vi "log analysis_gps.vi"() -> ()   [LabVIEW 2019] (continued)
8.2238,22.3000,0.0031,0.0013,-0.0034,-0.411270923,-0.605029312,287.914838543,0.2104,0.1573,0.2657,0.0344,0.0343,0.0312,0.0795,0.0805,4.9275,0f000005,0*6d07f4f4\n\t", "INSPVAXA,USB3,0,44.0,FINESTEERING,2107,283111.250,02000000,471d,15824;INS_ALIGNMENT_COMPLETE,INS_RTKFIXED,37.37108787798,126.72336901339,8.2237,22.3000,0.0035,0.0008,-0.0027,-0.411014484,-0.606801614,287.916144015,0.2104,0.1572,0.2653,0.0344,0.0343,0.0312,0.0795,0.0805,4.9290,0f000005,0*17fda63e\n\t", "INSPVAXA,USB3,0,46.5,FINESTEERING,2107,283112.250,02000000,471d,15824;INS_ALIGNMENT_COMPLETE,INS_RTKFIXED,37.37108788668,126.72336900523,8.2241,22.3000,0.0049,-0.0005,-0.0016,-0.408777501,-0.612185293,287.914677114,0.2103,0.1572,0.2649,0.0344,0.0343,0.0312,0.0795,0.0805,4.9305,0f000005,0*82ade194\n\t", "INSPVAXA,USB3,0,46.5,FINESTEERING,2107,283112.750,02000000,471d,15824;INS_ALIGNMENT_COMPLETE,INS_RTKFIXED,37.37108788778,126.72336899951,8.2242,22.3000,0.0047,-0.0009,-0.0019,-0.409122282,-0.611972311,287.914890224,0.2103,0.1572,0.2649,0.0344,0.0343,0.0312,0.0795,0.0805,4.9305,0f000005,0*c3a4b162\n\t", "INSPVAXA,USB3,0,48.5,FINESTEERING,2107,283113.250,02000000,471d,15824;INS_ALIGNMENT_COMPLETE,INS_RTKFIXED,37.37108788861,126.72336899425,8.2243,22.3000,0.0050,-0.0013,-0.0019,-0.410508140,-0.611024198,287.914176571,0.2103,0.1572,0.2646,0.0344,0.0343,0.0312,0.0795,0.0805,4.9321,0f000005,0*87d2d5b6\n\t", "INSPVAXA,USB3,0,48.5,FINESTEERING,2107,283113.750,02000000,471d,15824;INS_ALIGNMENT_COMPLETE,INS_RTKFIXED,37.37108789363,126.72336898840,8.2244,22.3000,0.0063,-0.0021,-0.0017,-0.411022705,-0.609051513,287.913579305,0.2103,0.1572,0.2646,0.0344,0.0343,0.0312,0.0795,0.0805,4.9321,0f000005,0*35e79e67\n\t", "INSPVAXA,USB3,0,47.0,FINESTEERING,2107,283114.250,02000000,471d,15824;INS_ALIGNMENT_COMPLETE,INS_RTKFIXED,37.37108789523,126.72336898295,8.2245,22.3000,0.0061,-0.0024,-0.0023,-0.410389175,-0.608679796,287.908436695,0.2102,0.1572,0.2643,0.0344,0.0343,0.0312,0.0795,0.0805,4.9336,0f000005,0*e900128e\n\t", "INSPVAXA,USB3,0,47.0,FINESTEERING,2107,283114.750,02000000,471d,15824;INS_ALIGNMENT_COMPLETE,INS_RTKFIXED,37.37108789043,126.72336897889,8.2245,22.3000,0.0054,-0.0027,-0.0027,-0.410079836,-0.608000188,287.907030910,0.2102,0.1572,0.2643,0.0344,0.0343,0.0312,0.0795,0.0805,4.9336,0f000005,0*f5aa2bf4\n\t", "INSPVAXA,USB3,0,46.0,FINESTEERING,2107,283115.250,02000000,471d,15824;INS_ALIGNMENT_COMPLETE,INS_RTKFIXED,37.37108788786,126.72336897498,8.2245,22.3000,0.0055,-0.0029,-0.0021,-0.409736809,-0.602715261,287.905938302,0.2101,0.1572,0.2640,0.0344,0.0343,0.0312,0.0795,0.0805,4.9352,0f000005,0*b8856e6c\n\t", "INSPVAXA,USB3,0,46.0,FINESTEERING,2107,283115.750,02000000,471d,15824;INS_ALIGNMENT_COMPLETE,INS_RTKFIXED,37.37108788493,126.72336897577,8.2245,22.3000,0.0046,-0.0023,-0.0026,-0.410098984,-0.602405796,287.902959038,0.2101,0.1572,0.2640,0.0344,0.0343,0.0312,0.0795,0.0805,4.9352,0f000005,0*5724c76a\n\t", "INSPVAXA,USB3,0,48.5,FINESTEERING,2107,283117.250,02000000,471d,15824;INS_ALIGNMENT_COMPLETE,INS_RTKFIXED,37.37108787822,126.72336898248,8.2247,22.3000,0.0046,0.0006,-0.0022,-0.408932053,-0.597708499,287.898385765,0.2100,0.1572,0.2634,0.0344,0.0343,0.0312,0.0795,0.0805,4.9381,0f000005,0*450763d8\n\t", "INSPVAXA,USB3,0,51.5,FINESTEERING,2107,283118.750,02000000,471d,15824;INS_ALIGNMENT_COMPLETE,INS_RTKFIXED,37.37108787489,126.72336898888,8.2255,22.3000,0.0051,0.0006,-0.0004,-0.410553255,-0.597325999,287.895855349,0.2099,0.1572,0.2632,0.0344,0.0343,0.0312,0.0794,0.0805,4.9396,0f000005,0*531bbf8e\n\t", "INSPVAXA,USB3,0,49.0,FINESTEERING,2107,283119.750,02000000,471d,15824;INS_ALIGNMENT_COMPLETE,INS_RTKFIXED,37.37108788239,126.72336898736,8.2256,22.3000,0.0062,0.0005,-0.0005,-0.410245690,-0.596223685,287.896349306,0.2099,0.1572,0.2630,0.0344,0.0343,0.0312,0.0794,0.0805,4.9410,0f000005,0*aabca186\n\t", "INSPVAXA,USB3,0,47.5,FINESTEERING,2107,283120.250,02000000,471d,15824;INS_ALIGNMENT_COMPLETE,INS_RTKFIXED,37.37108788462,126.72336898711,8.2255,22.3000,0.0062,0.0002,-0.0014,-0.410019875,-0.596819628,287.894466218,0.2099,0.1572,0.2628,0.0344,0.0343,0.0312,0.0794,0.0805,4.9425,0f000005,0*feb71611\n\t", "INSPVAXA,USB3,0,47.5,FINESTEERING,2107,283121.250,02000000,471d,15824;INS_ALIGNMENT_COMPLETE,INS_RTKFIXED,37.37108788020,126.72336899019,8.2251,22.3000,0.0049,0.0012,-0.0017,-0.410504520,-0.596359600,287.895045223,0.2098,0.1572,0.2627,0.0344,0.0343,0.0312,0.0794,0.0805,4.9439,0f000005,0*861abdab\n\t", "INSPVAXA,USB3,0,48.0,FINESTEERING,2107,283122.250,02000000,471d,15824;INS_ALIGNMENT_COMPLETE,INS_RTKFIXED,37.37108788140,126.72336898679,8.2256,22.3000,0.0046,0.0003,-0.0020,-0.412214067,-0.597500472,287.894257245,0.2098,0.1572,0.2625,0.0344,0.0343,0.0312,0.0794,0.0805,4.9454,0f000005,0*41de74d7\n\t", "INSPVAXA,USB3,0,46.5,FINESTEERING,2107,283126.250,02000000,471d,15824;INS_ALIGNMENT_COMPLETE,INS_RTKFIXED,37.37108785781,126.72336899407,8.2263,22.3000,0.0034,0.0010,-0.0014,-0.405163325,-0.599911050,287.885200973,0.2098,0.1572,0.2620,0.0344,0.0343,0.0312,0.0794,0.0804,4.9511,0f000005,0*554930fc\n\t", "INSPVAXA,USB3,0,50.5,FINESTEERING,2107,283133.250,02008000,471d,15824;INS_ALIGNMENT_COMPLETE,INS_RTKFIXED,37.37108787441,126.72336901696,8.2251,22.3000,0.0051,0.0025,0.0013,-0.401038405,-0.592309574,287.886306258,0.2098,0.1572,0.2615,0.0344,0.0343,0.0312,0.0794,0.0804,4.9611,0f000005,0*3f736d45\n\t", "INSPVAXA,USB3,0,50.0,FINESTEERING,2107,283145.800,02000000,471d,15824;INS_ALIGNMENT_COMPLETE,INS_RTKFIXED,37.37108786440,126.72336901151,8.2210,22.3000,0.0034,-0.0002,0.0004,-0.408176107,-0.602369941,287.881922019,0.2098,0.1572,0.2612,0.0344,0.0343,0.0312,0.0794,0.0804,4.9785,0f000005,0*1b1c4bf8\n\t", "INSPVAXA,USB3,0,45.5,FINESTEERING,2107,283151.800,02000000,471d,15824;INS_ALIGNMENT_COMPLETE,INS_RTKFIXED,37.37108787046,126.72336898866,8.2212,22.3000,0.0033,0.0009,-0.0006,-0.404916149,-0.597406910,287.865620586,0.2099,0.1572,0.2612,0.0344,0.0343,0.0312,0.0793,0.0804,4.9878,0f000005,0*a5f125e6\n\t", "INSPVAXA,USB3,0,45.0,FINESTEERING,2107,283152.300,02000000,471d,15824;INS_ALIGNMENT_COMPLETE,INS_RTKFIXED,37.37108786806,126.72336899217,8.2208,22.3000,0.0029,0.0018,-0.0009,-0.404359469,-0.596798726,287.864856489,0.2099,0.1572,0.2612,0.0344,0.0343,0.0312,0.0793,0.0804,4.9892,0f000005,0*75438a82\n\t", "INSPVAXA,USB3,0,47.5,FINESTEERING,2107,283153.800,02000000,471d,15824;INS_ALIGNMENT_COMPLETE,INS_RTKFIXED,37.37108786600,126.72336899902,8.2205,22.3000,0.0026,0.0021,-0.0023,-0.403425682,-0.598266477,287.862635982,0.2098,0.1572,0.2612,0.0344,0.0343,0.0312,0.0793,0.0804,4.9906,0f000005,0*5c2a9c66\n\t", "INSPVAXA,USB3,0,49.0,FINESTEERING,2107,283155.800,02000000,471d,15824;INS_ALIGNMENT_COMPLETE,INS_RTKFIXED,37.37108786878,126.72336899361,8.2202,22.3000,0.0032,0.0004,-0.0022,-0.395795579,-0.599014783,287.862450492,0.2098,0.1572,0.2612,0.0344,0.0343,0.0312,0.0793,0.0804,4.9935,0f000005,0*f4cd5051\n\t", "INSPVAXA,USB3,0,46.5,FINESTEERING,2107,283156.300,02000000,471d,15824;INS_ALIGNMENT_COMPLETE,INS_RTKFIXED,37.37108786919,126.72336899093,8.2205,22.3000,0.0038,-0.0001,-0.0013,-0.396437672,-0.598313647,287.862503112,0.2098,0.1572,0.2612,0.0344,0.0343,0.0312,0.0793,0.0804,4.9950,0f000005,0*5aa32664\n\t", "INSPVAXA,USB3,0,46.5,FINESTEERING,2107,283156.800,02000000,471d,15824;INS_ALIGNMENT_COMPLETE,INS_RTKFIXED,37.37108787385,126.72336898941,8.2207,22.3000,0.0043,-0.0002,-0.0010,-0.392731293,-0.598638690,287.862042656,0.2098,0.1572,0.2612,0.0344,0.0343,0.0312,0.0793,0.0804,4.9950,0f000005,0*03d612e4\n\t", "INSPVAXA,USB3,0,51.0,FINESTEERING,2107,283157.300,02000000,471d,15824;INS_ALIGNMENT_COMPLETE,INS_RTKFIXED,37.37108787685,126.72336898846,8.2211,22.3000,0.0052,-0.0002,-0.0000,-0.390778583,-0.597437105,287.863000385,0.2098,0.1573,0.2612,0.0344,0.0343,0.0312,0.0793,0.0804,4.9965,0f000005,0*3bc0d928\n\t", "INSPVAXA,USB3,0,50.5,FINESTEERING,2107,283159.300,02000000,471d,15824;INS_ALIGNMENT_COMPLETE,INS_RTKFIXED,37.37108788569,126.72336899544,8.2223,22.3000,0.0068,0.0019,0.0013,-0.387086330,-0.593973069,287.861144002,0.2098,0.1573,0.2612,0.0344,0.0343,0.0312,0.0793,0.0803,4.9994,0f000005,0*0ed095af\n\t", "INSPVAXA,USB3,0,44.5,FINESTEERING,2107,283160.800,02000000,471d,15824;INS_ALIGNMENT_COMPLETE,INS_RTKFIXED,37.37108790025,126.72336900642,8.2224,22.3000,0.0087,0.0034,0.0012,-0.385305357,-0.593887975,287.861236180,0.2098,0.1573,0.2612,0.0344,0.0343,0.0312,0.0793,0.0803,5.0008,0f000005,0*a535fac5\n\t", "INSPVAXA,USB3,0,47.0,FINESTEERING,2107,283161.800,02000000,471d,15824;INS_ALIGNMENT_COMPLETE,INS_RTKFIXED,37.37108791058,126.72336901739,8.2224,22.3000,0.0091,0.0053,0.0008,-0.384677214,-0.593155644,287.863440186,0.2098,0.1573,0.2612,0.0344,0.0343,0.0312,0.0793,0.0803,5.0020,0f000005,0*15bd2f54\n\t", "INSPVAXA,USB3,0,49.0,FINESTEERING,2107,283162.300,02000000,471d,15824;INS_ALIGNMENT_COMPLETE,INS_RTKFIXED,37.37108791275,126.72336902289,8.2223,22.3000,0.0092,0.0053,0.0006,-0.383976052,-0.593983766,287.863552246,0.2098,0.1573,0.2612,0.0344,0.0343,0.0312,0.0793,0.0803,5.0033,0f000005,0*f7f4aafb\n\t", "INSPVAXA,USB3,0,49.0,FINESTEERING,2107,283162.800,02000000,471d,15824;INS_ALIGNMENT_COMPLETE,INS_RTKFIXED,37.37108791707,126.72336902756,8.2221,22.3000,0.0099,0.0052,0.0004,-0.383244439,-0.593582797,287.863703162,0.2098,0.1573,0.2612,0.0344,0.0343,0.0312,0.0793,0.0803,5.0033,0f000005,0*87119b1a\n\t", "INSPVAXA,USB3,0,50.0,FINESTEERING,2107,283163.300,02000000,471d,15824;INS_ALIGNMENT_COMPLETE,INS_RTKFIXED,37.37108791768,126.72336903031,8.2218,22.3000,0.0093,0.0052,-0.0002,-0.382087992,-0.594481290,287.864257970,0.2098,0.1573,0.2612,0.0344,0.0343,0.0312,0.0793,0.0803,5.0046,0f000005,0*64efd3fe\n\t", "INSPVAXA,USB3,0,50.0,FINESTEERING,2107,283163.800,02000000,471d,15824;INS_ALIGNMENT_COMPLETE,INS_RTKFIXED,37.37108791823,126.72336903544,8.2213,22.3000,0.0087,0.0054,-0.0002,-0.381855357,-0.594537838,287.865100598,0.2098,0.1573,0.2612,0.0344,0.0343,0.0312,0.0793,0.0803,5.0046,0f000005,0*eaa89ec3\n\t", "INSPVAXA,USB3,0,49.5,FINESTEERING,2107,283164.300,02000000,471d,15824;INS_ALIGNMENT_COMPLETE,INS_RTKFIXED,37.37108791762,126.72336903818,8.2211,22.3000,0.0096,0.0053,-0.0000,-0.380427968,-0.595358698,287.865754120,0.2100,0.1573,0.2613,0.0344,0.0343,0.0312,0.0793,0.0803,5.0060,0f000005,0*9eb07253\n\t", "INSPVAXA,USB3,0,49.5,FINESTEERING,2107,283164.800,02000000,471d,15824;INS_ALIGNMENT_COMPLETE,INS_RTKFIXED,37.37108792129,126.72336904200,8.2211,22.3000,0.0095,0.0050,0.0001,-0.381479450,-0.593246291,287.867192627,0.2100,0.1573,0.2613,0.0344,0.0343,0.0312,0.0793,0.0803,5.0060,0f000005,0*81097ed9\n\t", "INSPVAXA,USB3,0,48.5,FINESTEERING,2107,283165.300,02000000,471d,15824;INS_ALIGNMENT_COMPLETE,INS_RTKFIXED,37.37108792359,126.72336904372,8.2212,22.3000,0.0098,0.0050,0.0003,-0.382461437,-0.592905475,287.870739528,0.2103,0.1573,0.2614,0.0344,0.0343,0.0312,0.0793,0.0803,5.0073,0f000005,0*f350cda0\n\t", "INSPVAXA,USB3,0,48.5,FINESTEERING,2107,283165.800,02000000,471d,15824;INS_ALIGNMENT_COMPLETE,INS_RTKFIXED,37.37108792768,126.72336904655,8.2215,22.3000,0.0096,0.0053,0.0004,-0.381584283,-0.591456419,287.872579847,0.2103,0.1573,0.2614,0.0344,0.0343,0.0312,0.0793,0.0803,5.0073,0f000005,0*a9ef8806\n\t", "INSPVAXA,USB3,0,47.0,FINESTEERING,2107,283166.300,02000000,471d,15824;INS_ALIGNMENT_COMPLETE,INS_RTKFIXED,37.37108793024,126.72336904905,8.2215,22.3000,0.0104,0.0057,0.0003,-0.382222726,-0.592164318,287.872646767,0.2105,0.1573,0.2615,0.0344,0.0343,0.0312,0.0793,0.0803,5.0087,0f000005,0*6f064ef0\n\t", "INSPVAXA,USB3,0,47.0,FINESTEERING,2107,283166.800,02000000,471d,15824;INS_ALIGNMENT_COMPLETE,INS_RTKFIXED,37.37108793672,126.72336905212,8.2216,22.3000,0.0107,0.0058,0.0001,-0.380800259,-0.589429313,287.874913684,0.2105,0.1573,0.2615,0.0344,0.0343,0.0312,0.0793,0.0803,5.0087,0f000005,0*ee96ecc4\n\t", "INSPVAXA,USB3,0,48.0,FINESTEERING,2107,283167.300,02000000,471d,15824;INS_ALIGNMENT_COMPLETE,INS_RTKFIXED,37.37108797180,126.72336907746,8.2214,22.3000,0.0123,0.0072,-0.0009,-0.380175638,-0.588519598,287.873648229,0.2105,0.1573,0.2615,0.0344,0.0343,0.0312,0.0793,0.0803,5.0087,0f000005,0*c5785aa0\n\t", "INSPVAXA,USB3,0,48.0,FINESTEERING,2107,283167.800,02000000,471d,15824;INS_ALIGNMENT_COMPLETE,INS_RTKFIXED,37.37108803292,126.72336912346,8.2209,22.3000,0.0149,0.0089,-0.0014,-0.377171042,-0.586737055,287.872482646,0.2105,0.1573,0.2615,0.0344,0.0343,0.0312,0.0793,0.0803,5.0087,0f000005,0*c60ea973\n\t", "INSPVAXA,USB3,0,42.0,FINESTEERING,2107,283168.300,02000000,471d,15824;INS_ALIGNMENT_COMPLETE,INS_RTKFIXED,37.37108803880,126.72336912583,8.2209,22.3000,0.0161,0.0086,-0.0017,-0.375595415,-0.586259403,287.874300642,0.2244,0.1729,0.2724,0.0385,0.0383,0.0343,0.0796,0.0805,5.0113,0f000005,0*8044c93c\n\t", "INSPVAXA,USB3,0,42.0,FINESTEERING,2107,283168.800,02000000,471d,15824;INS_ALIGNMENT_COMPLETE,INS_RTKFIXED,37.37108800795,126.72336909694,8.2215,22.3000,0.0141,0.0074,-0.0014,-0.380382564,-0.586190595,287.878476093,0.2244,0.1729,0.2724,0.0385,0.0383,0.0343,0.0796,0.0805,5.0113,0f000005,0*54eab961\n\t", "INSPVAXA,USB3,0,47.5,FINESTEERING,2107,283169.300,02000000,471d,15824;INS_ALIGNMENT_COMPLETE,INS_RTKFIXED,37.37108798474,126.72336907996,8.2218,22.3000,0.0121,0.0069,-0.0018,-0.383839466,-0.586517581,287.881593098,0.2239,0.1710,0.2714,0.0357,0.0355,0.0323,0.0788,0.0798,5.0127,0f000005,0*36e8c713\n\t", "INSPVAXA,USB3,0,47.5,FINESTEERING,2107,283169.800,02000000,471d,15824;INS_ALIGNMENT_COMPLETE,INS_RTKFIXED,37.37108797168,126.72336907326,8.2216,22.3000,0.0108,0.0060,-0.0021,-0.382641749,-0.586060307,287.885088335,0.2239,0.1710,0.2714,0.0357,0.0355,0.0323,0.0788,0.0798,5.0127,0f000005,0*d441264a\n\t", "INSPVAXA,USB3,0,49.5,FINESTEERING,2107,283170.300,02000000,471d,15824;INS_ALIGNMENT_COMPLETE,INS_RTKFIXED,37.37108796269,126.72336906818,8.2217,22.3000,0.0104,0.0055,-0.0014,-0.383475872,-0.583542182,287.889042259,0.2231,0.1689,0.2708,0.0348,0.0347,0.0316,0.0786,0.0797,5.0142,0f000005,0*32689bb7\n\t", "INSPVAXA,USB3,0,49.5,FINESTEERING,2107,283170.800,02000000,471d,15824;INS_ALIGNMENT_COMPLETE,INS_RTKFIXED,37.37108796102,126.72336906813,8.2219,22.3000,0.0104,0.0056,-0.0013,-0.382678847,-0.583610963,287.888842190,0.2231,0.1689,0.2708,0.0348,0.0347,0.0316,0.0786,0.0797,5.0142,0f000005,0*5e85f202\n\t", "INSPVAXA,USB3,0,48.5,FINESTEERING,2107,283171.300,02000000,471d,15824;INS_ALIGNMENT_COMPLETE,INS_RTKFIXED,37.37108796031,126.72336906830,8.2221,22.3000,0.0098,0.0065,-0.0020,-0.382671205,-0.583618137,287.888068003,0.2220,0.1670,0.2703,0.0345,0.0344,0.0314,0.0786,0.0797,5.0156,0f000005,0*d6c1e6dd\n\t", "INSPVAXA,USB3,0,48.5,FINESTEERING,2107,283171.800,02000000,471d,15824;INS_ALIGNMENT_COMPLETE,INS_RTKFIXED,37.37108796545,126.72336907471,8.2220,22.3000,0.0105,0.0071,-0.0022,-0.380415359,-0.582586820,287.889750442,0.2220,0.1670,0.2703,0.0345,0.0344,0.0314,0.0786,0.0797,5.0156,0f000005,0*ca9dcfb0\n\t", "INSPVAXA,USB3,0,50.0,FINESTEERING,2107,283172.300,02000000,471d,15824;INS_ALIGNMENT_COMPLETE,INS_RTKFIXED,37.37108796771,126.72336907645,8.2222,22.3000,0.0108,0.0068,-0.0016,-0.379539912,-0.580787545,287.890138856,0.2209,0.1652,0.2698,0.0344,0.0343,0.0313,0.0787,0.0798,5.0170,0f000005,0*259de970\n\t", "INSPVAXA,USB3,0,50.0,FINESTEERING,2107,283172.800,02000000,471d,15824;INS_ALIGNMENT_COMPLETE,INS_RTKFIXED,37.37108797403,126.72336907678,8.2227,22.3000,0.0110,0.0071,-0.0014,-0.379066228,-0.579747038,287.892022667,0.2209,0.1652,0.2698,0.0344,0.0343,0.0313,0.0787,0.0798,5.0170,0f000005,0*0ecf865b\n\t", "INSPVAXA,USB3,0,51.5,FINESTEERING,2107,283173.300,02000000,471d,15824;INS_ALIGNMENT_COMPLETE,INS_RTKFIXED,37.37108801209,126.72336910611,8.2226,22.3000,0.0136,0.0085,-0.0010,-0.377696334,-0.579038466,287.894073906,0.2209,0.1652,0.2698,0.0344,0.0343,0.0313,0.0787,0.0798,5.0170,0f000005,0*92cf69d3\n\t", "INSPVAXA,USB3,0,51.5,FINESTEERING,2107,283173.800,02000000,471d,15824;INS_ALIGNMENT_COMPLETE,INS_RTKFIXED,37.37108808085,126.72336916289,8.2221,22.3000,0.0168,0.0112,-0.0008,-0.373536353,-0.577127426,287.890111312,0.2209,0.1652,0.2698,0.0344,0.0343,0.0313,0.0787,0.0798,5.0170,0f000005,0*81360348\n\t", "DUALANTENNAHEADINGA,USB3,0,44.0,FINESTEERING,2107,283174.300,02000000,d426,15824;INSUFFICIENT_OBS,NONE,-1.000000000,0.000000000,0.000000000,0.0,0.000000000,0.000000000,\"631T\",17,4,4,3,04,00,20,03*70a0cfeb\n\t", "DUALANTENNAHEADINGA,USB3,0,44.0,FINESTEERING,2107,283174.800,02000000,d426,15824;INSUFFICIENT_OBS,NONE,-1.000000000,0.000000000,0.000000000,0.0,0.000000000,0.000000000,\"631T\",15,4,4,3,04,00,20,03*9126eb2e\n\t", "DUALANTENNAHEADINGA,USB3,0,49.0,FINESTEERING,2107,283175.300,02000000,d426,15824;INSUFFICIENT_OBS,NONE,-1.000000000,0.000000000,0.000000000,0.0,0.000000000,0.000000000,\"631T\",14,2,2,2,04,00,20,00*c59d9589\n\t", "INSPVAXA,USB3,0,49.0,FINESTEERING,2107,283175.800,02000000,471d,15824;INS_ALIGNMENT_COMPLETE,INS_RTKFIXED,37.37108802047,126.72336911665,8.2237,22.3000,0.0129,0.0096,0.0019,-0.378938573,-0.573397489,287.902596878,0.2314,0.1754,0.2784,0.0357,0.0355,0.0323,0.0784,0.0795,5.0209,0f000005,0*65843865\n\t", "INSPVAXA,USB3,0,50.0,FINESTEERING,2107,283176.300,02000000,471d,15824;INS_ALIGNMENT_COMPLETE,INS_RTKFIXED,37.37108801184,126.72336911067,8.2239,22.3000,0.0121,0.0095,0.0018,-0.379072967,-0.575586336,287.905355097,0.2295,0.1724,0.2772,0.0348,0.0346,0.0316,0.0783,0.0794,5.0222,0f000005,0*c18ce629\n\t", "INSPVAXA,USB3,0,50.0,FINESTEERING,2107,283176.800,02000000,471d,15824;INS_ALIGNMENT_COMPLETE,INS_RTKFIXED,37.37108800756,126.72336910969,8.2238,22.3000,0.0114,0.0095,0.0012,-0.381926010,-0.578081656,287.907841439,0.2295,0.1724,0.2772,0.0348,0.0346,0.0316,0.0783,0.0794,5.0222,0f000005,0*ef194e5b\n\t", "DUALANTENNAHEADINGA,USB3,0,49.0,FINESTEERING,2107,283177.300,02000000,d426,15824;INSUFFICIENT_OBS,NONE,-1.000000000,0.000000000,0.000000000,0.0,0.000000000,0.000000000,\"631T\",17,2,2,2,04,00,20,00*bd7b1a92\n\t", "DUALANTENNAHEADINGA,USB3,0,49.0,FINESTEERING,2107,283177.800,02000000,d426,15824;INSUFFICIENT_OBS,NONE,-1.000000000,0.000000000,0.000000000,0.0,0.000000000,0.000000000,\"631T\",16,2,2,2,04,00,20,00*ffabb8fe\n\t", "DUALANTENNAHEADINGA,USB3,0,48.5,FINESTEERING,2107,283178.300,02000000,d426,15824;INSUFFICIENT_OBS,NONE,-1.000000000,0.000000000,0.000000000,0.0,0.000000000,0.000000000,\"631T\",16,2,2,2,04,00,20,00*59fc98a6\n\t", "INSPVAXA,USB3,0,48.5,FINESTEERING,2107,283178.800,02000000,471d,15824;INS_ALIGNMENT_COMPLETE,INS_RTKFIXED,37.37108800752,126.72336911614,8.2234,22.3000,0.0091,0.0098,0.0003,-0.383716997,-0.576517366,287.910600308,0.2256,0.1673,0.2752,0.0344,0.0343,0.0313,0.0786,0.0797,5.0251,0f000005,0*a6696e29\n\t", "DUALANTENNAHEADINGA,USB3,0,49.5,FINESTEERING,2107,283179.300,02000000,d426,15824;INSUFFICIENT_OBS,NONE,-1.000000000,0.000000000,0.000000000,0.0,0.000000000,0.000000000,\"631T\",12,2,2,2,04,00,20,00*b9084739\n\t", "INSPVAXA,USB3,0,49.5,FINESTEERING,2107,283179.800,02000000,471d,15824;INS_ALIGNMENT_COMPLETE,INS_RTKFIXED,37.37108800248,126.72336912231,8.2230,22.3000,0.0076,0.0089,-0.0004,-0.383606530,-0.576962847,287.915737403,0.2238,0.1653,0.2743,0.0344,0.0342,0.0313,0.0787,0.0798,5.0265,0f000005,0*ee90b331\n\t", "INSPVAXA,USB3,0,48.5,FINESTEERING,2107,283180.300,02000000,471d,15824;INS_ALIGNMENT_COMPLETE,INS_RTKFIXED,37.37108799880,126.72336912044,8.2230,22.3000,0.0074,0.0084,-0.0003,-0.382763287,-0.577609398,287.917624770,0.2223,0.1637,0.2735,0.0344,0.0342,0.0312,0.0788,0.0799,5.0279,0f000005,0*b9fcfa2d\n\t", "DUALANTENNAHEADINGA,USB3,0,48.5,FINESTEERING,2107,283180.800,02000000,d426,15824;INSUFFICIENT_OBS,NONE,-1.000000000,0.000000000,0.000000000,0.0,0.000000000,0.000000000,\"631T\",14,2,2,2,04,00,20,00*67370902\n\t", "INSPVAXA,USB3,0,51.0,FINESTEERING,2107,283181.300,02000000,471d,15824;INS_ALIGNMENT_COMPLETE,INS_RTKFIXED,37.37108799142,126.72336911584,8.2227,22.3000,0.0062,0.0073,-0.0012,-0.379070208,-0.579479951,287.919184058,0.2209,0.1624,0.2727,0.0344,0.0342,0.0312,0.0789,0.0800,5.0294,0f000005,0*ff5c7a42\n\t", "INSPVAXA,USB3,0,51.0,FINESTEERING,2107,283181.800,02000000,471d,15824;INS_ALIGNMENT_COMPLETE,INS_RTKFIXED,37.37108798938,126.72336911647,8.2229,22.3000,0.0064,0.0075,-0.0013,-0.378914786,-0.582250994,287.920027881,0.2209,0.1624,0.2727,0.0344,0.0342,0.0312,0.0789,0.0800,5.0294,0f000005,0*210c1369\n\t", "INSPVAXA,USB3,0,50.5,FINESTEERING,2107,283182.300,02000000,471d,15824;INS_ALIGNMENT_COMPLETE,INS_RTKFIXED,37.37108798784,126.72336911574,8.2231,22.3000,0.0069,0.0073,-0.0014,-0.376950030,-0.581137760,287.919196566,0.2197,0.1614,0.2720,0.0344,0.0342,0.0312,0.0790,0.0800,5.0308,0f000005,0*5d6efddc\n\t", "INSPVAXA,USB3,0,50.5,FINESTEERING,2107,283182.800,02000000,471d,15824;INS_ALIGNMENT_COMPLETE,INS_RTKFIXED,37.37108799276,126.72336911883,8.2233,22.3000,0.0080,0.0075,-0.0014,-0.377644437,-0.581747143,287.919278227,0.2197,0.1614,0.2720,0.0344,0.0342,0.0312,0.0790,0.0800,5.0308,0f000005,0*2c1378c7\n\t", "INSPVAXA,USB3,0,50.0,FINESTEERING,2107,283183.300,02000000,471d,15824;INS_ALIGNMENT_COMPLETE,INS_RTKFIXED,37.37108799440,126.72336911810,8.2235,22.3000,0.0083,0.0077,-0.0003,-0.377907999,-0.580976107,287.918524275,0.2187,0.1605,0.2713,0.0344,0.0342,0.0312,0.0791,0.0801,5.0323,0f000005,0*3971cbaa\n\t", "DUALANTENNAHEADINGA,USB3,0,50.0,FINESTEERING,2107,283183.800,02000000,d426,15824;INSUFFICIENT_OBS,NONE,-1.000000000,0.000000000,0.000000000,0.0,0.000000000,0.000000000,\"631T\",15,2,2,2,04,00,20,00*16dcf878\n\t", "INSPVAXA,USB3,0,49.5,FINESTEERING,2107,283184.300,02000000,471d,15824;INS_ALIGNMENT_COMPLETE,INS_RTKFIXED,37.37108799290,126.72336911350,8.2241,22.3000,0.0072,0.0062,0.0001,-0.380085189,-0.579242316,287.919684164,0.2178,0.1599,0.2707,0.0344,0.0343,0.0312,0.0792,0.0801,5.0339,0f000005,0*bc5fd1df\n\t", "DUALANTENNAHEADINGA,USB3,0,49.5,FINESTEERING,2107,283184.800,02000000,d426,15824;INSUFFICIENT_OBS,NONE,-1.000000000,0.000000000,0.000000000,0.0,0.000000000,0.000000000,\"631T\",15,2,2,2,04,00,20,00*b8804adb\n\t", "INSPVAXA,USB3,0,51.0,FINESTEERING,2107,283185.300,02000000,471d,15824;INS_ALIGNMENT_COMPLETE,INS_RTKFIXED,37.37108798957,126.72336910890,8.2243,22.3000,0.0072,0.0065,0.0004,-0.376376594,-0.581358564,287.922376317,0.2170,0.1594,0.2701,0.0344,0.0343,0.0312,0.0792,0.0802,5.0354,0f000005,0*e79d958c\n\t", "DUALANTENNAHEADINGA,USB3,0,51.0,FINESTEERING,2107,283185.800,02000000,d426,15824;INSUFFICIENT_OBS,NONE,-1.000000000,0.000000000,0.000000000,0.0,0.000000000,0.000000000,\"631T\",15,2,2,2,04,00,20,00*c539324b\n\t", "INSPVAXA,USB3,0,49.5,FINESTEERING,2107,283186.300,02000000,471d,15824;INS_ALIGNMENT_COMPLETE,INS_RTKFIXED,37.37108798620,126.72336910856,8.2243,22.3000,0.0071,0.0073,-0.0002,-0.377506910,-0.583623217,287.927831882,0.2163,0.1590,0.2696,0.0344,0.0343,0.0312,0.0792,0.0802,5.0369,0f000005,0*21523d82\n\t", "DUALANTENNAHEADINGA,USB3,0,49.5,FINESTEERING,2107,283186.800,02000000,d426,15824;INSUFFICIENT_OBS,NONE,-1.000000000,0.000000000,0.000000000,0.0,0.000000000,0.000000000,\"631T\",14,4,4,3,04,00,20,03*758328f4\n\t", "INSPVAXA,USB3,0,46.0,FINESTEERING,2107,283187.300,02000000,471d,15824;INS_ALIGNMENT_COMPLETE,INS_RTKFIXED,37.37108798055,126.72336910974,8.2240,22.3000,0.0067,0.0070,0.0001,-0.381669916,-0.586056120,287.928395893,0.2158,0.1586,0.2691,0.0344,0.0343,0.0312,0.0793,0.0802,5.0384,0f000005,0*68985769\n\t", "INSPVAXA,USB3,0,46.0,FINESTEERING,2107,283187.800,02000000,471d,15824;INS_ALIGNMENT_COMPLETE,INS_RTKFIXED,37.37108797480,126.72336910787,8.2241,22.3000,0.0056,0.0073,-0.0002,-0.384514938,-0.587125643,287.930034096,0.2158,0.1586,0.2691,0.0344,0.0343,0.0312,0.0793,0.0802,5.0384,0f000005,0*a7c7a978\n\t", "DUALANTENNAHEADINGA,USB3,0,50.5,FINESTEERING,2107,283188.300,02000000,d426,15824;INSUFFICIENT_OBS,NONE,-1.000000000,0.000000000,0.000000000,0.0,0.000000000,0.000000000,\"631T\",15,2,2,2,04,00,20,00*b8de1ba1\n\t", "INSPVAXA,USB3,0,50.5,FINESTEERING,2107,283188.800,02000000,471d,15824;INS_ALIGNMENT_COMPLETE,INS_RTKFIXED,37.37108796465,126.72336910438,8.2240,22.3000,0.0044,0.0069,-0.0006,-0.384553588,-0.585982152,287.932075352,0.2153,0.1584,0.2687,0.0344,0.0343,0.0312,0.0793,0.0802,5.0398,0f000005,0*584615a0\n\t", "DUALANTENNAHEADINGA,USB3,0,50.0,FINESTEERING,2107,283189.300,02008000,d426,15824;SOL_COMPUTED,L1_FLOAT,-1.000000000,22.943321228,-27.912841797,0.0,360.000000000,180.000000000,\"631T\",17,5,5,3,04,00,20,03*61e408ae\n\t", "INSPVAXA,USB3,0,50.0,FINESTEERING,2107,283189.800,02008000,471d,15824;INS_ALIGNMENT_COMPLETE,INS_RTKFIXED,37.37108795686,126.72336910595,8.2245,22.3000,0.0035,0.0080,-0.0003,-0.386062307,-0.585594940,287.936481773,0.2149,0.1582,0.2683,0.0344,0.0343,0.0312,0.0793,0.0802,5.0412,0f000005,0*927e0823\n\t", "DUALANTENNAHEADINGA,USB3,0,46.5,FINESTEERING,2107,283190.300,02008000,d426,15824;SOL_COMPUTED,L1_FLOAT,-1.000000000,295.270263672,43.260082245,0.0,360.000000000,180.000000000,\"631T\",14,5,5,3,04,00,20,03*6a966b3f\n\t", "DUALANTENNAHEADINGA,USB3,0,46.5,FINESTEERING,2107,283190.800,02008000,d426,15824;SOL_COMPUTED,L1_FLOAT,-1.000000000,350.638061523,5.315610409,0.0,360.000000000,180.000000000,\"631T\",13,5,5,3,04,00,20,03*8fee928e\n\t", "DUALANTENNAHEADINGA,USB3,0,51.0,FINESTEERING,2107,283191.300,02008000,d426,15824;SOL_COMPUTED,L1_FLOAT,-1.000000000,12.310025215,-18.113586426,0.0,360.000000000,180.000000000,\"631T\",14,5,5,3,04,00,20,03*cb2a916c\n\t", "DUALANTENNAHEADINGA,USB3,0,51.0,FINESTEERING,2107,283191.800,02008000,d426,15824;SOL_COMPUTED,L1_FLOAT,-1.000000000,35.111301422,-35.377624512,0.0,101.695205688,180.000000000,\"631T\",14,5,5,3,04,00,20,03*191bd153\n\t", "INSPVAXA,USB3,0,48.0,FINESTEERING,2107,283192.300,02008000,471d,15824;INS_ALIGNMENT_COMPLETE,INS_RTKFIXED,37.37108795667,126.72336911311,8.2256,22.3000,0.0046,0.0093,0.0005,-0.387858319,-0.587901427,287.938370105,0.2139,0.1579,0.2673,0.0344,0.0343,0.0312,0.0793,0.0802,5.0456,0f000005,0*318753ed\n\t", "DUALANTENNAHEADINGA,USB3,0,48.0,FINESTEERING,2107,283192.800,02008000,d426,15824;SOL_COMPUTED,L1_FLOAT,-1.000000000,28.920713425,-31.830932617,0.0,228.720611572,180.000000000,\"631T\",14,5,5,3,04,00,20,03*dfadfb53\n\t", "DUALANTENNAHEADINGA,USB3,0,52.5,FINESTEERING,2107,283193.300,02008000,d426,15824;SOL_COMPUTED,L1_FLOAT,-1.000000000,22.577627182,-27.194854736,0.0,360.000000000,180.000000000,\"631T\",14,5,5,3,04,00,20,03*2b92c623\n\t", "INSPVAXA,USB3,0,52.5,FINESTEERING,2107,283193.800,02008000,471d,15824;INS_ALIGNMENT_COMPLETE,INS_RTKFIXED,37.37108794696,126.72336913145,8.2245,22.3000,0.0046,0.0096,-0.0011,-0.386759073,-0.585024800,287.941284128,0.2137,0.1578,0.2670,0.0344,0.0343,0.0312,0.0793,0.0802,5.0469,0f000005,0*303171d6\n\t", "INSPVAXA,USB3,0,47.5,FINESTEERING,2107,283194.300,02008000,471d,15824;INS_ALIGNMENT_COMPLETE,INS_RTKFIXED,37.37108794768,126.72336913167,8.2241,22.3000,0.0062,0.0083,-0.0013,-0.387313384,-0.586457322,287.941677020,0.2135,0.1577,0.2667,0.0344,0.0343,0.0312,0.0793,0.0802,5.0484,0f000005,0*fb34fba9\n\t", "DUALANTENNAHEADINGA,USB3,0,47.5,FINESTEERING,2107,283194.800,02008000,d426,15824;SOL_COMPUTED,L1_FLOAT,-1.000000000,15.914994240,-22.873901367,0.0,360.000000000,180.000000000,\"631T\",14,5,5,3,04,00,20,03*a57ffdb4\n\t", "DUALANTENNAHEADINGA,USB3,0,50.5,FINESTEERING,2107,283195.300,02008000,d426,15824;INSUFFICIENT_OBS,NONE,-1.000000000,0.000000000,0.000000000,0.0,0.000000000,0.000000000,\"631T\",14,4,4,4,04,00,20,20*483b483f\n\t", "DUALANTENNAHEADINGA,USB3,0,50.5,FINESTEERING,2107,283195.800,02008000,d426,15824;INSUFFICIENT_OBS,NONE,-1.000000000,0.000000000,0.000000000,0.0,0.000000000,0.000000000,\"631T\",16,4,4,4,04,00,20,20*a9bd6cfa\n\t", "DUALANTENNAHEADINGA,USB3,0,48.5,FINESTEERING,2107,283196.300,02008000,d426,15824;INSUFFICIENT_OBS,NONE,-1.000000000,0.000000000,0.000000000,0.0,0.000000000,0.000000000,\"631T\",16,4,4,4,04,00,20,20*cffcd920\n\t", "DUALANTENNAHEADINGA,USB3,0,48.5,FINESTEERING,2107,283196.800,02008000,d426,15824;INSUFFICIENT_OBS,NONE,-1.000000000,0.000000000,0.000000000,0.0,0.000000000,0.000000000,\"631T\",16,4,4,4,04,00,20,20*5acefb14\n\t", "DUALANTENNAHEADINGA,USB3,0,49.0,FINESTEERING,2107,283197.300,02008000,d426,15824;INSUFFICIENT_OBS,NONE,-1.000000000,0.000000000,0.000000000,0.0,0.000000000,0.000000000,\"631T\",16,4,4,4,04,00,20,20*931aed91\n\t", "DUALANTENNAHEADINGA,USB3,0,49.0,FINESTEERING,2107,283197.800,02008000,d426,15824;INSUFFICIENT_OBS,NONE,-1.000000000,0.000000000,0.000000000,0.0,0.000000000,0.000000000,\"631T\",16,4,4,4,04,00,20,20*0628cfa5\n\t", "DUALANTENNAHEADINGA,USB3,0,48.5,FINESTEERING,2107,283198.300,02000000,d426,15824;SOL_COMPUTED,L1_FLOAT,-1.000000000,255.227523804,12.823373795,0.0,360.000000000,180.000000000,\"631T\",14,5,5,4,04,00,20,03*2801eac2\n\t", "DUALANTENNAHEADINGA,USB3,0,48.5,FINESTEERING,2107,283198.800,02000000,d426,15824;SOL_COMPUTED,L1_FLOAT,-1.000000000,26.448829651,-49.172851563,0.0,283.970214844,136.538162231,\"631T\",14,5,5,4,04,00,20,03*767a920f\n\t", "DUALANTENNAHEADINGA,USB3,0,48.5,FINESTEERING,2107,283199.300,02000000,d426,15824;INSUFFICIENT_OBS,NONE,-1.000000000,0.000000000,0.000000000,0.0,0.000000000,0.000000000,\"631T\",15,4,4,3,04,00,20,03*ae2edc4c\n\t", "DUALANTENNAHEADINGA,USB3,0,48.5,FINESTEERING,2107,283199.800,02000000,d426,15824;INSUFFICIENT_OBS,NONE,-1.000000000,0.000000000,0.000000000,0.0,0.000000000,0.000000000,\"631T\",16,4,4,3,04,00,20,03*984a78d1\n\t", "DUALANTENNAHEADINGA,USB3,0,47.0,FINESTEERING,2107,283200.300,02000000,d426,15824;INSUFFICIENT_OBS,NONE,-1.000000000,0.000000000,0.000000000,0.0,0.000000000,0.000000000,\"631T\",14,4,4,3,04,00,20,03*7a2c4abd\n\t", "DUALANTENNAHEADINGA,USB3,0,47.0,FINESTEERING,2107,283200.800,02000000,d426,15824;INSUFFICIENT_OBS,NONE,-1.000000000,0.000000000,0.000000000,0.0,0.000000000,0.000000000,\"631T\",14,4,4,3,04,00,20,03*ef1e6889\n\t", "DUALANTENNAHEADINGA,USB3,0,50.0,FINESTEERING,2107,283201.300,02000000,d426,15824;INSUFFICIENT_OBS,NONE,-1.000000000,0.000000000,0.000000000,0.0,0.000000000,0.000000000,\"631T\",15,2,2,2,04,00,20,00*363721e3\n\t", "DUALANTENNAHEADINGA,USB3,0,50.0,FINESTEERING,2107,283201.800,02000000,d426,15824;INSUFFICIENT_OBS,NONE,-1.000000000,0.000000000,0.000000000,0.0,0.000000000,0.000000000,\"631T\",16,2,2,2,04,00,20,00*0053857e\n\t", "DUALANTENNAHEADINGA,USB3,0,47.5,FINESTEERING,2107,283202.300,02000000,d426,15824;INSUFFICIENT_OBS,NONE,-1.000000000,0.000000000,0.000000000,0.0,0.000000000,0.000000000,\"631T\",15,2,2,2,04,00,20,00*e255ce5e\n\t", "DUALANTENNAHEADINGA,USB3,0,47.5,FINESTEERING,2107,283202.800,02000000,d426,15824;INSUFFICIENT_OBS,NONE,-1.000000000,0.000000000,0.000000000,0.0,0.000000000,0.000000000,\"631T\",14,2,2,2,04,00,20,00*a0856c32\n\t", "DUALANTENNAHEADINGA,USB3,0,48.5,FINESTEERING,2107,283203.300,02000000,d426,15824;INSUFFICIENT_OBS,NONE,-1.000000000,0.000000000,0.000000000,0.0,0.000000000,0.000000000,\"631T\",16,2,2,2,04,00,20,00*5eb0d2b1\n\t", "DUALANTENNAHEADINGA,USB3,0,48.5,FINESTEERING,2107,283203.800,02000000,d426,15824;INSUFFICIENT_OBS,NONE,-1.000000000,0.000000000,0.000000000,0.0,0.000000000,0.000000000,\"631T\",16,2,2,2,04,00,20,00*cb82f085\n\t", "DUALANTENNAHEADINGA,USB3,0,47.5,FINESTEERING,2107,283204.300,02000000,d426,15824;INSUFFICIENT_OBS,NONE,-1.000000000,0.000000000,0.000000000,0.0,0.000000000,0.000000000,\"631T\",18,2,2,2,04,00,20,00*62df42f6\n\t", "DUALANTENNAHEADINGA,USB3,0,47.5,FINESTEERING,2107,283204.800,02000000,d426,15824;INSUFFICIENT_OBS,NONE,-1.000000000,0.000000000,0.000000000,0.0,0.000000000,0.000000000,\"631T\",17,2,2,2,04,00,20,00*b472f60c\n\t", "DUALANTENNAHEADINGA,USB3,0,46.5,FINESTEERING,2107,283205.300,02000000,d426,15824;INSUFFICIENT_OBS,NONE,-1.000000000,0.000000000,0.000000000,0.0,0.000000000,0.000000000,\"631T\",15,2,2,2,04,00,20,00*5c6800b4\n\t", "DUALANTENNAHEADINGA,USB3,0,46.5,FINESTEERING,2107,283205.800,02000000,d426,15824;INSUFFICIENT_OBS,NONE,-1.000000000,0.000000000,0.000000000,0.0,0.000000000,0.000000000,\"631T\",15,2,2,2,04,00,20,00*c95a2280\n\t", "DUALANTENNAHEADINGA,USB3,0,49.0,FINESTEERING,2107,283206.300,02000000,d426,15824;INSUFFICIENT_OBS,NONE,-1.000000000,0.000000000,0.000000000,0.0,0.000000000,0.000000000,\"631T\",14,2,2,2,04,00,20,00*1af3f5d4\n\t", "DUALANTENNAHEADINGA,USB3,0,49.0,FINESTEERING,2107,283206.800,02000000,d426,15824;INSUFFICIENT_OBS,NONE,-1.000000000,0.000000000,0.000000000,0.0,0.000000000,0.000000000,\"631T\",13,2,2,2,04,00,20,00*c5ff5cab\n\t", "DUALANTENNAHEADINGA,USB3,0,49.5,FINESTEERING,2107,283207.300,02000000,d426,15824;INSUFFICIENT_OBS,NONE,-1.000000000,0.000000000,0.000000000,0.0,0.000000000,0.000000000,\"631T\",12,2,2,2,04,00,20,00*bf8d1cd2\n\t", "DUALANTENNAHEADINGA,USB3,0,49.5,FINESTEERING,2107,283207.800,02000000,d426,15824;INSUFFICIENT_OBS,NONE,-1.000000000,0.000000000,0.000000000,0.0,0.000000000,0.000000000,\"631T\",12,2,2,2,04,00,20,00*2abf3ee6\n\t", "DUALANTENNAHEADINGA,USB3,0,47.0,FINESTEERING,2107,283208.300,02000000,d426,15824;INSUFFICIENT_OBS,NONE,-1.000000000,0.000000000,0.000000000,0.0,0.000000000,0.000000000,\"631T\",14,4,4,3,04,00,20,03*a20e60f7\n\t", "DUALANTENNAHEADINGA,USB3,0,47.0,FINESTEERING,2107,283208.800,02000000,d426,15824;INSUFFICIENT_OBS,NONE,-1.000000000,0.000000000,0.000000000,0.0,0.000000000,0.000000000,\"631T\",15,4,4,3,04,00,20,03*e0dec29b\n\t", "DUALANTENNAHEADINGA,USB3,0,47.5,FINESTEERING,2107,283209.300,02000000,d426,15824;INSUFFICIENT_OBS,NONE,-1.000000000,0.000000000,0.000000000,0.0,0.000000000,0.000000000,\"631T\",14,4,4,3,04,00,20,03*9aac82e2\n\t", "INSPVAXA,USB3,0,47.5,FINESTEERING,2107,283209.850,02000000,471d,15824;INS_ALIGNMENT_COMPLETE,INS_RTKFIXED,37.37108793670,126.72336902912,8.2230,22.3000,0.0057,0.0015,0.0021,-0.400587739,-0.588760253,287.923723239,0.2124,0.1575,0.2644,0.0344,0.0343,0.0312,0.0792,0.0802,5.0715,0f000005,0*2296f550\n\t", "DUALANTENNAHEADINGA,USB3,0,44.5,FINESTEERING,2107,283211.300,02000000,d426,15824;INSUFFICIENT_OBS,NONE,-1.000000000,0.000000000,0.000000000,0.0,0.000000000,0.000000000,\"631T\",14,4,4,3,04,00,20,03*11216130\n\t", "DUALANTENNAHEADINGA,USB3,0,44.5,FINESTEERING,2107,283211.800,02000000,d426,15824;INSUFFICIENT_OBS,NONE,-1.000000000,0.000000000,0.000000000,0.0,0.000000000,0.000000000,\"631T\",17,4,4,3,04,00,20,03*2745c5ad\n\t", "DUALANTENNAHEADINGA,USB3,0,48.0,FINESTEERING,2107,283212.800,02000000,d426,15824;INSUFFICIENT_OBS,NONE,-1.000000000,0.000000000,0.000000000,0.0,0.000000000,0.000000000,\"631T\",17,4,4,3,04,00,20,03*1af1cb79\n\t", "DUALANTENNAHEADINGA,USB3,0,47.5,FINESTEERING,2107,283213.300,02000000,d426,15824;INSUFFICIENT_OBS,NONE,-1.000000000,0.000000000,0.000000000,0.0,0.000000000,0.000000000,\"631T\",17,4,4,3,04,00,20,03*c50a95c7\n\t", "INSPVAXA,USB3,0,47.5,FINESTEERING,2107,283213.850,02000000,471d,15824;INS_ALIGNMENT_COMPLETE,INS_RTKFIXED,37.37108793573,126.72336903807,8.2229,22.3000,0.0072,0.0033,-0.0007,-0.395561271,-0.586256352,287.924343856,0.2123,0.1575,0.2642,0.0344,0.0343,0.0312,0.0792,0.0802,5.0774,0f000005,0*129510f9\n\t", "INSPVAXA,USB3,0,49.0,FINESTEERING,2107,283214.350,02000000,471d,15824;INS_ALIGNMENT_COMPLETE,INS_RTKFIXED,37.37108793342,126.72336903992,8.2230,22.3000,0.0065,0.0039,-0.0008,-0.396825161,-0.583976103,287.925419134,0.2123,0.1575,0.2641,0.0344,0.0343,0.0312,0.0792,0.0802,5.0789,0f000005,0*b5398675\n\t", "DUALANTENNAHEADINGA,USB3,0,49.0,FINESTEERING,2107,283214.800,02000000,d426,15824;INSUFFICIENT_OBS,NONE,-1.000000000,0.000000000,0.000000000,0.0,0.000000000,0.000000000,\"631T\",14,4,4,3,04,00,20,03*6a4287e3\n\t", "DUALANTENNAHEADINGA,USB3,0,48.5,FINESTEERING,2107,283215.300,02000000,d426,15824;INSUFFICIENT_OBS,NONE,-1.000000000,0.000000000,0.000000000,0.0,0.000000000,0.000000000,\"631T\",17,4,4,3,04,00,20,03*00c017cf\n\t", "DUALANTENNAHEADINGA,USB3,0,48.5,FINESTEERING,2107,283215.800,02000000,d426,15824;INSUFFICIENT_OBS,NONE,-1.000000000,0.000000000,0.000000000,0.0,0.000000000,0.000000000,\"631T\",16,4,4,3,04,00,20,03*4210b5a3\n\t", "DUALANTENNAHEADINGA,USB3,0,44.5,FINESTEERING,2107,283216.300,02000000,d426,15824;INSUFFICIENT_OBS,NONE,-1.000000000,0.000000000,0.000000000,0.0,0.000000000,0.000000000,\"631T\",16,4,4,3,04,00,20,03*bfec7f8f\n\t", "DUALANTENNAHEADINGA,USB3,0,49.5,FINESTEERING,2107,283217.300,02000000,d426,15824;INSUFFICIENT_OBS,NONE,-1.000000000,0.000000000,0.000000000,0.0,0.000000000,0.000000000,\"631T\",16,4,4,3,04,00,20,03*68d64881\n\t", "INSPVAXA,USB3,0,49.5,FINESTEERING,2107,283217.850,02000000,471d,15824;INS_ALIGNMENT_COMPLETE,INS_RTKFIXED,37.37108791854,126.72336906586,8.2236,22.3000,0.0038,0.0069,-0.0005,-0.397358519,-0.581659593,287.929077774,0.2122,0.1575,0.2640,0.0344,0.0343,0.0312,0.0792,0.0802,5.0831,0f000005,0*bf1b0ee9\n\t", "INSPVAXA,USB3,0,49.0,FINESTEERING,2107,283218.850,02000000,471d,15824;INS_ALIGNMENT_COMPLETE,INS_RTKFIXED,37.37108791456,126.72336907619,8.2236,22.3000,0.0037,0.0083,-0.0011,-0.397325323,-0.588631877,287.932091771,0.2122,0.1575,0.2639,0.0344,0.0343,0.0312,0.0792,0.0802,5.0844,0f000005,0*75bb9db3\n\t", "INSPVAXA,USB3,0,48.5,FINESTEERING,2107,283219.350,02000000,471d,15824;INS_ALIGNMENT_COMPLETE,INS_RTKFIXED,37.37108791216,126.72336907891,8.2235,22.3000,0.0033,0.0082,-0.0011,-0.397206354,-0.592415954,287.932797733,0.2122,0.1575,0.2639,0.0344,0.0343,0.0312,0.0792,0.0802,5.0858,0f000005,0*61ec993c\n\t", "DUALANTENNAHEADINGA,USB3,0,48.5,FINESTEERING,2107,283219.800,02000000,d426,15824;INSUFFICIENT_OBS,NONE,-1.000000000,0.000000000,0.000000000,0.0,0.000000000,0.000000000,\"631T\",12,4,4,3,04,00,20,03*1f4b872e\n\t", "INSPVAXA,USB3,0,49.5,FINESTEERING,2107,283220.350,02000000,471d,15824;INS_ALIGNMENT_COMPLETE,INS_RTKFIXED,37.37108790624,126.72336908505,8.2229,22.3000,0.0022,0.0079,-0.0019,-0.399821313,-0.599696922,287.937754794,0.2122,0.1575,0.2639,0.0344,0.0343,0.0312,0.0792,0.0802,5.0871,0f000005,0*02520bc5\n\t", "DUALANTENNAHEADINGA,USB3,0,49.5,FINESTEERING,2107,283220.800,02000000,d426,15824;INSUFFICIENT_OBS,NONE,-1.000000000,0.000000000,0.000000000,0.0,0.000000000,0.000000000,\"631T\",14,4,4,3,04,00,20,03*89ffa4d7\n\t", "INSPVAXA,USB3,0,50.0,FINESTEERING,2107,283221.350,02000000,471d,15824;INS_ALIGNMENT_COMPLETE,INS_RTKFIXED,37.37108790285,126.72336908925,8.2228,22.3000,0.0035,0.0061,-0.0019,-0.399017543,-0.601198983,287.941471827,0.2122,0.1575,0.2639,0.0344,0.0343,0.0312,0.0792,0.0802,5.0886,0f000005,0*62ae3a3c\n\t", "DUALANTENNAHEADINGA,USB3,0,50.0,FINESTEERING,2107,283221.800,02000000,d426,15824;INSUFFICIENT_OBS,NONE,-1.000000000,0.000000000,0.000000000,0.0,0.000000000,0.000000000,\"631T\",15,4,4,3,04,00,20,03*47e08abb\n\t", "INSPVAXA,USB3,0,45.5,FINESTEERING,2107,283222.350,02000000,471d,15824;INS_ALIGNMENT_COMPLETE,INS_RTKFIXED,37.37108790796,126.72336908471,8.2224,22.3000,0.0048,0.0047,-0.0019,-0.398683572,-0.604525422,287.944164472,0.2123,0.1575,0.2638,0.0344,0.0343,0.0312,0.0792,0.0802,5.0901,0f000005,0*5070a156\n\t", "DUALANTENNAHEADINGA,USB3,0,45.5,FINESTEERING,2107,283222.800,02000000,d426,15824;INSUFFICIENT_OBS,NONE,-1.000000000,0.000000000,0.000000000,0.0,0.000000000,0.000000000,\"631T\",14,4,4,3,04,00,20,03*8ce94816\n\t", "INSPVAXA,USB3,0,50.0,FINESTEERING,2107,283223.350,02000000,471d,15824;INS_ALIGNMENT_COMPLETE,INS_RTKFIXED,37.37108790821,126.72336907660,8.2226,22.3000,0.0055,0.0030,-0.0018,-0.398800774,-0.606505226,287.948554602,0.2123,0.1575,0.2638,0.0344,0.0343,0.0312,0.0792,0.0802,5.0917,0f000005,0*2b7dac3f\n\t", "DUALANTENNAHEADINGA,USB3,0,49.5,FINESTEERING,2107,283224.300,02000000,d426,15824;INSUFFICIENT_OBS,NONE,-1.000000000,0.000000000,0.000000000,0.0,0.000000000,0.000000000,\"631T\",16,4,4,3,04,00,20,03*04689537\n\t", "INSPVAXA,USB3,0,49.5,FINESTEERING,2107,283224.850,02000000,471d,15824;INS_ALIGNMENT_COMPLETE,INS_RTKFIXED,37.37108790871,126.72336906996,8.2222,22.3000,0.0045,0.0021,-0.0033,-0.398675673,-0.605186622,287.948531011,0.2123,0.1575,0.2638,0.0344,0.0343,0.0312,0.0792,0.0802,5.0933,0f000005,0*5d419d28\n\t", "INSPVAXA,USB3,0,47.0,FINESTEERING,2107,283225.350,02000000,471d,15824;INS_ALIGNMENT_COMPLETE,INS_RTKFIXED,37.37108790579,126.72336906833,8.2219,22.3000,0.0039,0.0019,-0.0038,-0.399713651,-0.605242342,287.947949852,0.2123,0.1575,0.2638,0.0344,0.0343,0.0312,0.0792,0.0802,5.0949,0f000005,0*a40dd195\n\t", "INSPVAXA,USB3,0,47.0,FINESTEERING,2107,283225.850,02000000,471d,15824;INS_ALIGNMENT_COMPLETE,INS_RTKFIXED,37.37108794475,126.72336891478,8.2224,22.3000,0.0658,-0.1833,-0.0010,-0.392923625,-0.435798491,288.066022775,0.2123,0.1575,0.2638,
